vi "DAQmx产生脉冲设置.vi"(8 "error in":errorcluster) -> (0 "error out":errorcluster, 3 "task out":refnum<k21>)   [LabVIEW 2010]
doc: "This VI configures a task.\n\nYour program typically should execute this configuration code only once. To use this code in a loop, use the DAQmx ClearTask VI in the same loop."
uses:
  <vilib>/DAQmx/create/channels.llb/DAQmx Create Channel (CO-Pulse Generation-Time).vi
  <vilib>/DAQmx/configure/timing.llb/DAQmx Timing (Implicit).vi
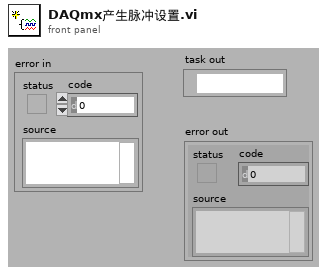
[diagram p1: front panel]
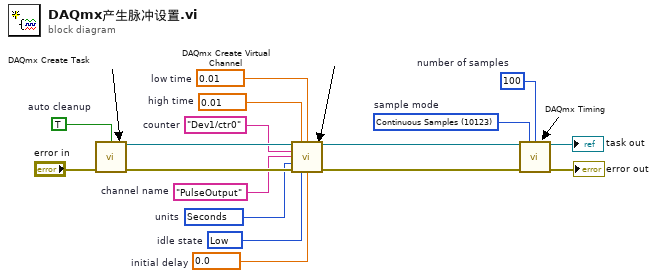
[diagram p0: block diagram]
diagram:
  w1 = 10123 items=["Finite Samples"=10178, "Continuous Samples"=10123]  # sample mode
  w2 = 100  # number of samples
  w5 = 0.01  # low time
  w6 = 0.01  # high time
  w7 = 0.0  # initial delay
  w8 = 10214 items=["High"=10192, "Low"=10214]  # idle state
  w9 = 10364 items=["Seconds"=10364, "From Custom Scale"=10065]  # units
  w10 = "PulseOutput"  # channel name
  w13 = "Dev1/ctr0"  # counter
  w14 = TRUE  # auto cleanup
  n1 = call <vilib>:"DAQmx Create Task.vi"("auto cleanup"=w14, "error in"="error in") -> ("task out"=w15:refnum<k21>, "error out"=w16:errorcluster)  [unwired: 12 in]
  n2 = call-poly <vilib>:"DAQmx Create Virtual Channel.vi"("task in"=w15, "high time"=w6, "low time"=w5, "counter"=w13, "name to assign"=w10, "units"=w9, "error in"=w16, "idle state"=w8, "initial delay"=w7) -> ("task out"=w12:refnum<k21>, "error out"=w11:errorcluster)  [unwired: 5 in]
  n3 = call-poly <vilib>:"DAQmx Timing.vi"("task/channels in"=w12, "sample mode"=w1, "samples per channel"=w2, "error in"=w11) -> ("task out"=→"task out":refnum<k21>, "error out"=→"error out":errorcluster)  [unwired: 10 in]
